vi "Set Ethernet IP.vi"(8 "Error In":errorcluster, 10 "IP Address":u32, 11 "LINX Device Config":T1) -> (0 "Error Out":errorcluster, 3 "LINX Device Config":T1)   [LabVIEW 2011, in "LVH-LINX.lvlib" / "Device.lvlib"]
doc: "Set the LINX device's ethernet IP address."
uses:
  Device.lvlib
  Type Defs/LINX Device Config.ctl
  Type Defs/Interface.ctl
  Type Defs/TCP Config.ctl
  Type Defs/Device Family.ctl
  Type Defs/Error Type.ctl
  LVH-LINX.lvlib
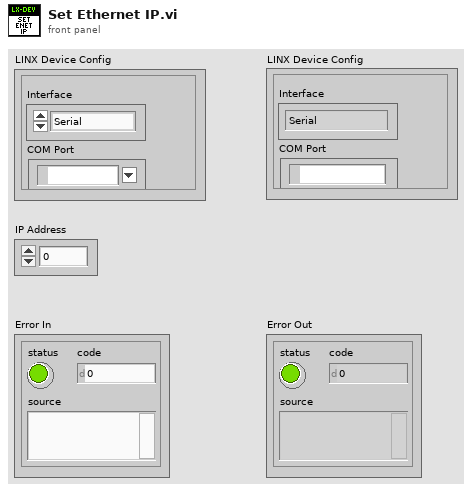
[diagram p1: front panel]
types:
  T1 = typedef "LVH-LINX.lvlib/Device.lvlib/LINX Device Config.ctl" = cluster{"Interface":T2, "COM Port":refnum<visa-resource-name>, "TCP Configuration":T3, "Device Family":T4, "Device ID":u8, "Device Name":string, "TCP Ref":refnum<k5>}
  T2 = typedef "LVH-LINX.lvlib/Interface.ctl" = enum16{"Serial", "TCP"}
  T3 = typedef "LVH-LINX.lvlib/Device.lvlib/TCP Config.ctl" = cluster{"IP Address":string, "Port":u16}
  T4 = typedef "LVH-LINX.lvlib/Device Family.ctl" = enum8{"National Instruments", "Digilent", "Arduino"}
  T5 = typedef "LVH-LINX.lvlib/Error Type.ctl" = enum16{"Unknown", "Timeout", "Corrupt Return Packet", "Unable To Connect", "Command Not Supported", "Channel DNE"}
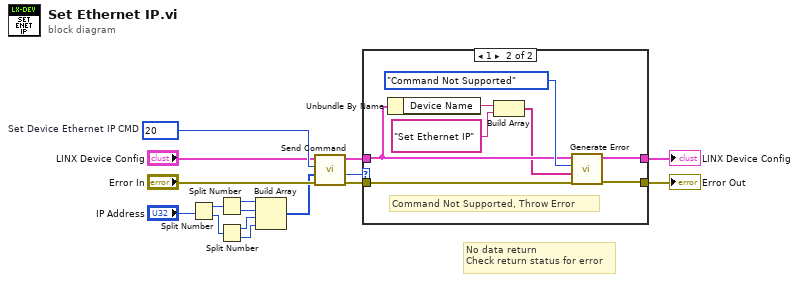
[diagram p0: block diagram]
diagram:
  w14 = u16 20  # Set Device Ethernet IP CMD
  # "No data return\nCheck return status for error"
  n1 = Split Number(x="IP Address") -> (hi(x)=w7:u16, lo(x)=w6:u16)
  n2 = Split Number(x=w7) -> (hi(x)=w5:u8, lo(x)=w4:u8)
  n3 = Split Number(x=w6) -> (hi(x)=w2:u8, lo(x)=w3:u8)
  n4 = Build Array(w5, w4, w2, w3) -> (w8:u8[])
  n5 = call "Send Command.vi"("Error In"="Error In", "ARGS"=w8, "CMD"=w14, "LINX Device Config"="LINX Device Config") -> ("Error Out"=w9:errorcluster, "Status"=w1:u8, "LINX Device Config"=w11:T1)  [unwired: 4 in, 1 out]
  n6 = case shown="1" w1 {
    tunnel: [w17 w24] -> w12
    tunnel: w11 -> [w17 w20]
    tunnel: [w18 w25] -> w10
    tunnel: w9 -> [w18 w26]
    frame 0, Default {
      # "Status OK, Process Data"
    }
    frame 1 {
      # "Command Not Supported, Throw Error"
      n7 = Unbundle By Name(w20) -> ("Device Name"=w21:string)
      n8 = Build Array(w21, "Set Ethernet IP") -> (w19:string[])
      n9 = call "Generate Error.vi"("Error In"=w26, "Arguments"=w19, "Error Type"=Error_Type."Command Not Supported", "LINX Device Config"=w20) -> ("Error Out"=w25:errorcluster, "LINX Device Config"=w24:T1)  [unwired: 6 in]
    }
  }
  "Error Out" <- w10
  "LINX Device Config" <- w12
